vi "CloseCurrentTree.vi"   [LabVIEW 2013]
uses:
  <vilib>/MDSplus/Library/MDSplus.lvlib
  <vilib>/MDSplus/Classes/Tree_Class/Tree.lvclass
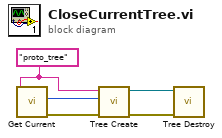
[diagram p0: block diagram]
diagram:
  w5 = "proto_tree" ("Name")
  n1 = call <vilib>:"Get Current.vi"("Tree name"=w5) -> ("error out"=w3:errorcluster, "Current shot out"=w4:i32)  [unwired: 8 in, 1 out]
  n2 = call <vilib>:"Tree Create.vi"("error in (no error)"=w3, "Shot"=w4, "Name"=w5) -> ("error out"=w1:errorcluster, "Tree DVR out"=w2:refnum<data-value>)  [unwired: 7 in]
  n3 = call <vilib>:"Tree Destroy.vi"("error in (no error)"=w1, "Tree DVR in"=w2) -> ()  [unwired: 9 in, 1 out]
